vi "Keithley J-t_IIT.vi"(4 "t step":dbl, 6 "V step":dbl, 7 "Sweep Direction":u16(ring) items=["Low to high", "High to low"], 8 "Measurement Delay (ms)":dbl=1.0, 9 "Max Voltage":dbl=2.0, 10 "MinVoltage":dbl=1.0, 11 "VISA resource name out 2":refnum<visa-resource-name>) -> (0 "Measurement Complete":bool, 2 "Data Array":dbl[][](array[numeric]), 3 "VISA resource name out":refnum<visa-resource-name>)   [LabVIEW 2011]
doc: "Configures a sweep and takes voltage and current readings at each point."
uses:
  <instrlib>/keithley_24xx/Keithley 24XX/Public/Data/Read (Single Point).vi
  <instrlib>/keithley_24xx/Keithley 24XX/Keithley 24XX.lvlib
panel:
  in  "Compliance  Level":dbl=0.1
  in  "Source Mode  (0: Voltage)":u16(ring) items=["Voltage", "Current"]
  # "(c) 2006 National Instruments.  ALL RIGHTS RESERVED."
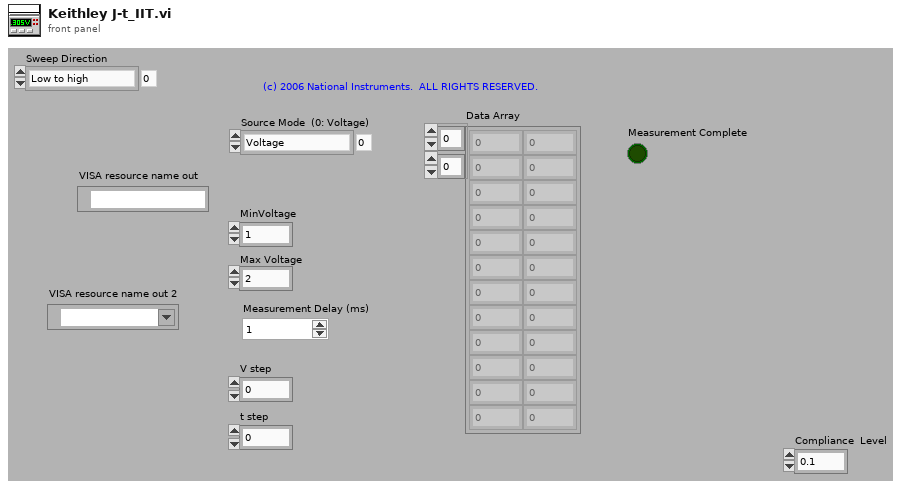
[diagram p1: front panel]
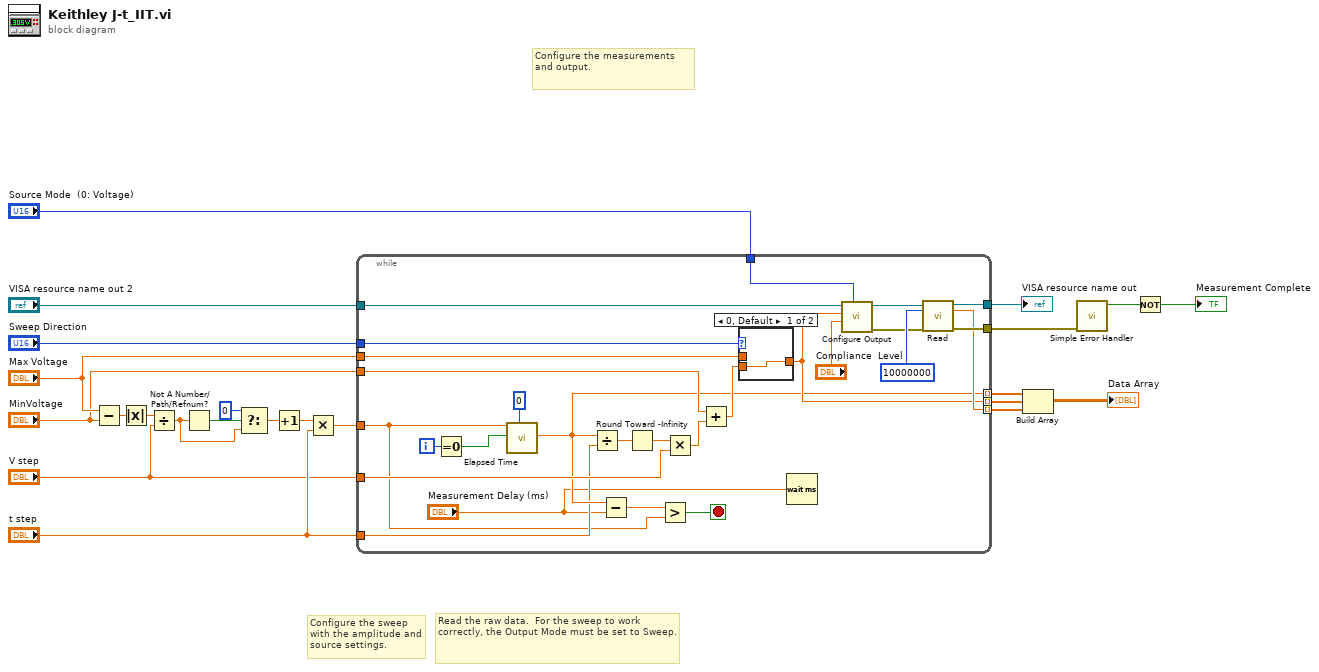
[diagram p0: block diagram]
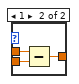
[diagram p2: hidden frame]
diagram:
  # "Read the raw data.  For the sweep to work correctly, the Output Mode must be set to Sweep."
  # "Configure the sweep with the amplitude and source settings."
  # "Configure the measurements and output."
  n1 = Subtract(x="Max Voltage", y="MinVoltage") -> (x-y=w2:dbl)
  n2 = Absolute Value(x=w2) -> (abs(x)=w3:dbl)
  n3 = Divide(x=w3, y="V step") -> (x/y=w16:dbl)
  n4 = Not A Number/Path/Refnum?(number/path/refnum=w16) -> (NaN/Path/Refnum?=w18:bool)
  n5 = Select(t=0, s=w18, f=w16) -> (s? t:f=w15:dbl)
  n6 = Increment(x=w15) -> (x+1=w14:dbl)
  n7 = Multiply(x=w14, y="t step") -> (x*y=w13:dbl)
  n8 = while {
    tunnel: [w50] -> w23
    tunnel: [w49] -> w22
    tunnel: w13 -> [w25]
    tunnel: "Source Mode  (0: Voltage)" -> [w44]
    tunnel: "VISA resource name out 2" -> [w43]
    tunnel: "t step" -> [w28]
    tunnel: "V step" -> [w40]
    tunnel: [w29] -> w9 mode=indexing
    tunnel: [w33] -> w8 mode=indexing
    tunnel: [w39] -> w7 mode=indexing
    tunnel: "Sweep Direction" -> [w38]
    tunnel: "Max Voltage" -> [w37]
    tunnel: "MinVoltage" -> [w34]
    i -> [w31]
    stop <- w27 stop-if-true
    n9 = Equal To 0?(x=w31) -> (x = 0?=w30:bool)
    n10 = call "Elapsed Time"("Time Target (s)"=w25, "Reset"=w30, "Set Start Time (s)"=0) -> ("Elapsed Time (s)"=w29:dbl)  [unwired: 9 in, 7 out]
    n11 = Divide(x=w29, y=w28) -> (x/y=w42:dbl)
    n12 = Subtract(x=w29, y="Measurement Delay (ms)") -> (x-y=w26:dbl)
    n13 = Round Toward -Infinity(1:w42) -> (0:w41:dbl)
    n14 = Greater?(x=w26, y=w25) -> (0:w27:bool)
    n15 = Multiply(x=w41, y=w40) -> (x*y=w36:dbl)
    n16 = Add(x=w34, y=w36) -> (x+y=w35:dbl)
    n17 = case shown="0, Default" w38 {
      tunnel: w37 -> [_ w54]
      tunnel: [w51 w53] -> w33
      tunnel: w35 -> [w51 w52]
      frame 0, Default {
      }
      frame 1 {
        n18 = Subtract(x=w54, y=w52) -> (x-y=w53:dbl)
      }
    }
    n19 = Wait (ms)(milliseconds to wait="Measurement Delay (ms)") -> ()  [unwired: 1 out]
    n20 = call <instrlib>:"Configure Output.vi"("Source Mode  (0: Voltage)"=w44, "Compliance  Level (0.1)"="Compliance  Level", "Output Level (0)"=w33, "VISA resource name"=w43) -> ("error out"=w46:errorcluster, "VISA resource name out"=w47:refnum<visa-resource-name>)  [unwired: 6 in]
    n21 = call-poly <instrlib>:"Read.vi"("VISA resource name"=w47, "Timeout (10000 ms)"=10000000, "error in (no error)"=w46) -> ("VISA resource name out"=w49:refnum<visa-resource-name>, "Current"=w39:sgl, "error out"=w50:errorcluster)  [unwired: 6 in, 4 out]
  }
  "VISA resource name out" <- w22
  n22 = Build Array(w9, w8, w7) -> (→"Data Array":dbl[][])
  n23 = call <vilib>:"Simple Error Handler.vi"("error in (no error)"=w23) -> ("error?"=w21:bool)  [unwired: 4 in, 4 out]
  n24 = Not(x=w21) -> (.not. x?=→"Measurement Complete":bool)
